vi "Values as Strings.vi"(8 "error in (no error)":errorcluster, 11 "Group in":refnum<class "Group.lvclass">) -> (0 "error out":errorcluster, 1 "Timestamps":dbl[](array[numeric]), 2 "Value Strings":string[](array[string]), 3 "Group out":refnum<class "Group.lvclass">)   [LabVIEW 2020, in "Vecto.lvlib" / "Group.lvclass"]
uses:
  Group.lvclass
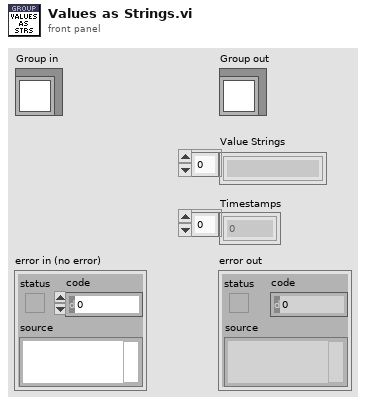
[diagram p1: front panel]
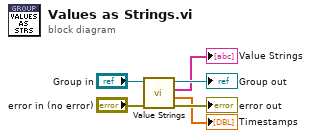
[diagram p0: block diagram]
diagram:
  n1 = call-dynamic "Value Strings.vi"("error in (no error)"="error in (no error)", "Group in"="Group in") -> ("error out"=→"error out":errorcluster, "Timestamp"=→"Timestamps":dbl[], "Value Strings"=→"Value Strings":string[], "Group out"=→"Group out":refnum<class "Group.lvclass">)  [unwired: 6 in]
